vi "initialise.vi"(8 "error in (no error)":errorcluster, 11 "GenericPlugin in":refnum<class "ImageAssemblerDL090211Scaffold.lvclass">) -> (0 "error out":errorcluster, 3 "GenericPlugin out":refnum<class "ImageAssemblerDL090211Scaffold.lvclass">)   [LabVIEW 2010, in "ImageAssemblerDL090211Scaffold.lvclass"]
doc: "The dynamic dispatch-version of this VI initalises the plug-in object by allocating and initalising any dynamic resources need."
uses:
  ImageAssemblerDL090211Scaffold.lvclass
  common/enumerations/top-level_component_type_enum.ctl
  GenericImageAssembler/GenericImageAssembler/GenericImageAssembler.lvclass
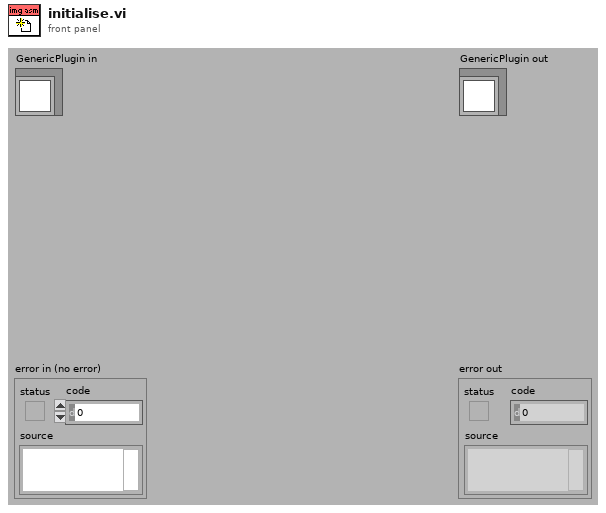
[diagram p1: front panel]
types:
  T1 = typedef "top-level_component_type_enum.ctl" = enum16{"undefined", "ImagingMode", "ScanHead", "DAQ", "ImageAssembler", "Display", "DataCollection", "Analyser", "Stimulator", "ExperimentController", "Instrument", "Stage"}
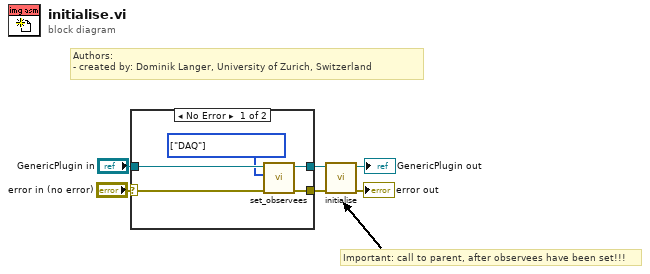
[diagram p0: block diagram]
diagram:
  # "Important: call to parent, after observees have been set!!!"
  # "Authors: \n- created by: Dominik Langer, University of Zurich, Switzerland"
  n1 = case shown="No Error" "error in (no error)" {
    selector: "error in (no error)" -> [w8 w13]
    tunnel: "GenericPlugin in" -> [w11 w12]
    tunnel: [w10 w12] -> w5
    tunnel: [w9 w13] -> w4
    frame No Error {
      w7 = T1[] [enum."DAQ"] items=["undefined", "ImagingMode", "ScanHead", "DAQ", "ImageAssembler", "Display", "DataCollection", "Analyser", "Stimulator", "ExperimentController", "Instrument", "Stage"] ("observees")
      n2 = call-dynamic "set_observees.vi"("error in (no error)"=w8, "observees"=w7, "GenericToplevelComponent in"=w11) -> ("error out"=w9:errorcluster, "GenericToplevelComponent out"=w10:refnum<class "ImageAssemblerDL090211Scaffold.lvclass">)  [unwired: 7 in]
    }
    frame Error {
    }
  }
  n3 = call-parent "initialise.vi"("error in (no error)"=w4, "GenericPlugin in"=w5) -> ("error out"=→"error out":errorcluster, "GenericPlugin out"=→"GenericPlugin out":refnum<class "ImageAssemblerDL090211Scaffold.lvclass">)  [unwired: 8 in]
